vi "Read Context Name.vi"(8 "error in (no error)":errorcluster, 11 "Server Config in":refnum<class "Server Config.lvclass">) -> (0 "error out":errorcluster, 2 "Context Name":string, 3 "Server Config out":refnum<class "Server Config.lvclass">)   [LabVIEW 2013, in "Server Controller.lvlib" / "Server Config.lvclass"]
uses:
  Server Config.lvclass
  Server Config.lvclass/Server Config.ctl
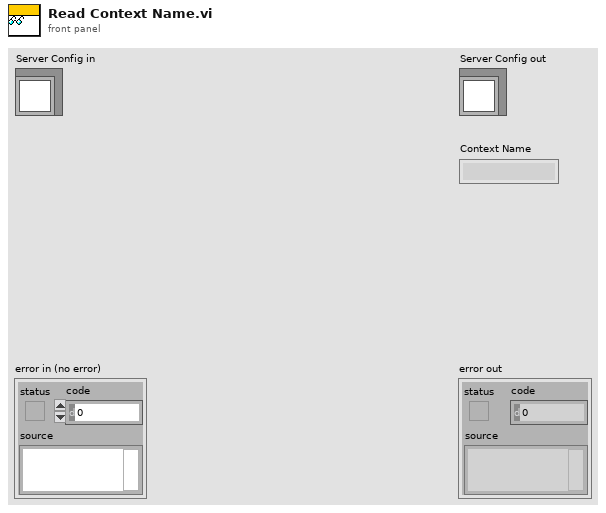
[diagram p1: front panel]
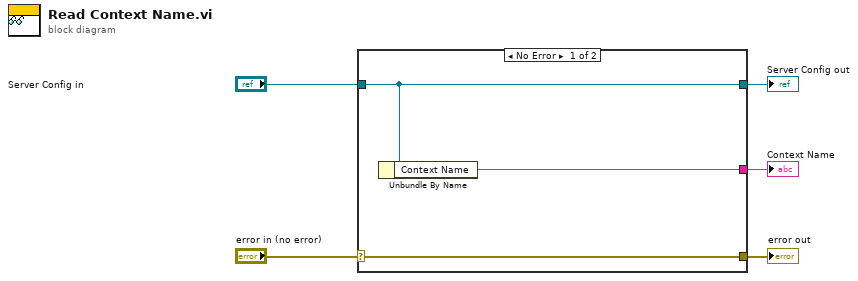
[diagram p0: block diagram]
diagram:
  n1 = case shown="No Error" "error in (no error)" {
    selector: "error in (no error)" -> [w8 w9]
    tunnel: [w8 w9] -> w4
    tunnel: [w7 w10] -> w2
    tunnel: "Server Config in" -> [w7 w10]
    tunnel: [w6 _] -> w1
    frame No Error {
      n2 = Unbundle By Name(w7) -> ("Context Name"=w6:string)
    }
    frame Error {
    }
  }
  "error out" <- w4
  "Server Config out" <- w2
  "Context Name" <- w1
